vi "Generic command handler.vi"(8 "error in (no error)":errorcluster, 10 "Message in":refnum<class "GenericMessage.lvclass">, 11 "BMC in":refnum<class "BMC.lvclass">) -> (0 "error out":errorcluster, 2 "value":string, 3 "BMC out":refnum<class "BMC.lvclass">)   [LabVIEW 2012, in "BMC.lvclass"]
doc: "The generic_command_handler processes the command 'generic'. Commands which are not part of the predefined list of commands fall under the 'generic' command for special activity."
uses:
  BMC.lvclass
  <vilib>/Distrio/Murmex/GenericMessage/GenericMessage.lvclass
  <vilib>/Distrio/Murmex/Murmex/Murmex.lvclass
  BMC.lvclass/BMC.ctl
panel:
  # "This method is called when the GENERIC\ntrigger is sent. \n\nOverride this method when your component needs to\nrespond to this trigger. \n\nCall parent for proper implementation"
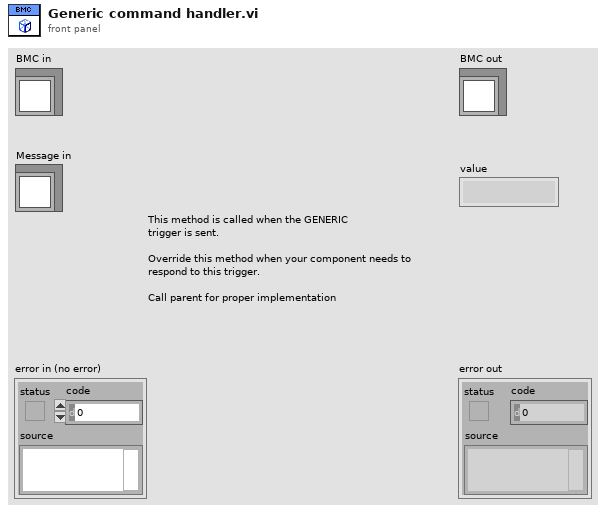
[diagram p1: front panel]
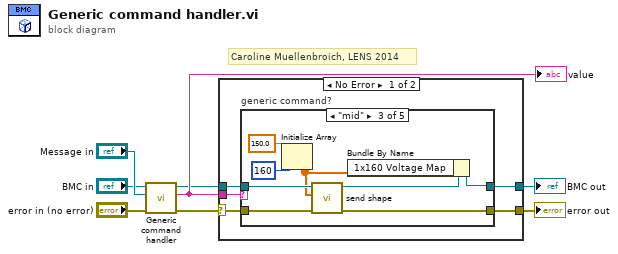
[diagram p0: block diagram]
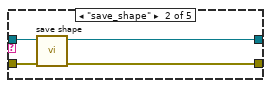
[diagram p3: hidden frame]
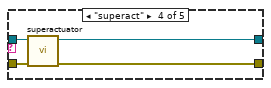
[diagram p4: hidden frame]
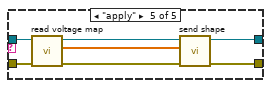
[diagram p5: hidden frame]
diagram:
  # "Caroline Muellenbroich, LENS 2014"
  n1 = call-parent "Generic command handler.vi"("error in (no error)"="error in (no error)", "Message in"="Message in", "Murmex in"="BMC in") -> ("error out"=w5:errorcluster, "value"=w4:string, "Murmex out"=w3:refnum<class "BMC.lvclass">)  [unwired: 6 in]
  "value" <- w4
  n2 = case shown="No Error" w5 {
    selector: w5 -> [w12 w39]
    tunnel: w4 -> [w13 _]
    tunnel: w3 -> [w9 w40]
    tunnel: [w11 w39] -> w2
    tunnel: [w10 w40] -> w1
    frame No Error {
      n3 = case "generic command?" shown="\"mid\"" w13 {
        tunnel: w12 -> [w14 w19 w26 w31 w38]
        tunnel: [w14 w18 w27 w30 w35] -> w11
        tunnel: [w15 w16 w20 w28 w36] -> w10
        tunnel: w9 -> [w15 w17 w25 w29 w37]
        frame Default {
        }
        frame "save_shape" {
          n4 = call-dynamic "save shape.vi"("error in (no error)"=w19, "BMC in"=w17) -> ("error out"=w18:errorcluster, "BMC out"=w16:refnum<class "BMC.lvclass">)  [unwired: 8 in]
        }
        frame "mid" {
          n5 = Initialize Array(150.0 ("element"), 160 ("dimension size")) -> (w22:dbl[])
          n6 = call-dynamic "send shape.vi"("error in (no error)"=w26, "1x160 Voltage Map"=w22, "BMC in"=w25) -> ("error out"=w27:errorcluster, "BMC out"=w21:refnum<class "BMC.lvclass">)  [unwired: 7 in]
          n7 = Bundle By Name(cluster=w21, "1x160 Voltage Map"=w22) -> (w20:refnum<class "BMC.lvclass">)
        }
        frame "superact" {
          n8 = call-dynamic "superactuator.vi"("error in (no error)"=w31, "BMC in"=w29) -> ("error out"=w30:errorcluster, "BMC out"=w28:refnum<class "BMC.lvclass">)  [unwired: 8 in]
        }
        frame "apply" {
          n9 = call-dynamic "read voltage map.vi"("error in (no error)"=w38, "BMC in"=w37) -> ("error out"=w32:errorcluster, "1x160 Voltage Map"=w33:dbl[], "BMC out"=w34:refnum<class "BMC.lvclass">)  [unwired: 7 in]
          n10 = call-dynamic "send shape.vi"("error in (no error)"=w32, "1x160 Voltage Map"=w33, "BMC in"=w34) -> ("error out"=w35:errorcluster, "BMC out"=w36:refnum<class "BMC.lvclass">)  [unwired: 7 in]
        }
      }
    }
    frame Error {
    }
  }
  "error out" <- w2
  "BMC out" <- w1
